vi "Sort moves by minimum incremental travel.vi"(1 "Coordinates to move through":sgl[][](array[numeric])) -> (0 "Indices sorted by minimum incremental travel distance":i32[](array[numeric]))   [LabVIEW 2014]
doc: "Sorts moves in order of minimum incremental linear travel distance, starting from the first point in the list."
uses:
  <vilib>/Analysis/baseanly.llb/Real Dot Product.vi
  <vilib>/Analysis/NI_AALBase.lvlib
panel:
  # "Paul Nathan 02/07/2015"
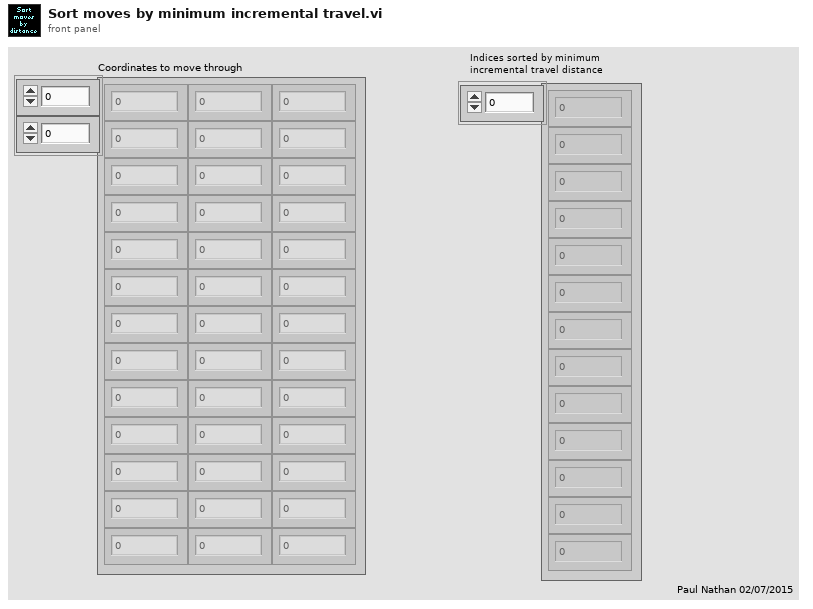
[diagram p1: front panel]
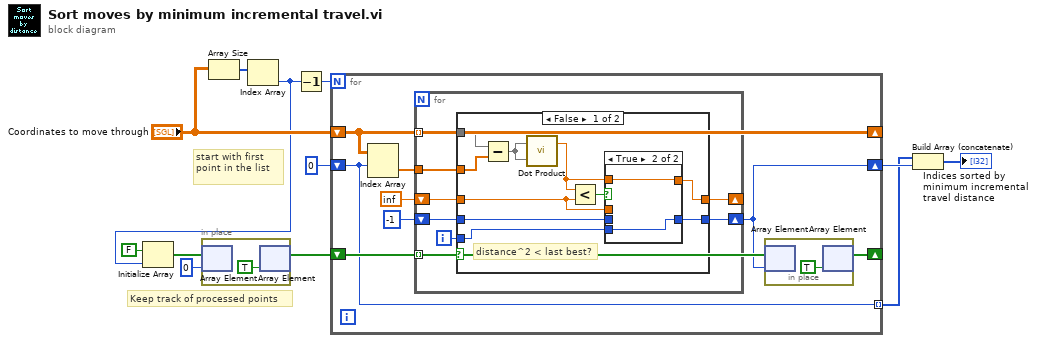
[diagram p0: block diagram]
diagram:
  # "Keep track of processed points"
  # "start with first point in the list"
  n1 = Array Size(array="Coordinates to move through") -> (size(s)=w11:i32[])
  n2 = Index Array(array=w11) -> (element=w9:i32)  [unwired: 1 in]
  n3 = Initialize Array(FALSE, w9) -> (w7:bool[])
  n4 = in-place {
    n5 = in-place-array #1(w7, 0) -> ()  [unwired: 1 out]
    n6 = in-place-array #1(TRUE ("element")) -> (w6:bool[])  [unwired: 1 out]
  }
  n7 = Decrement(x=w9) -> (x-1=w4:i32)
  n8 = for {
    N: w4 -> [_]
    shift-right: [w15] -> _
    shift-left: "Coordinates to move through" -> [w15]
    shift-right: [w19] -> _
    shift-left: w6 -> [w20]
    shift-right: [w16] -> w2
    shift-left: 0 -> [w14]
    tunnel: [w14] -> w1 mode=indexing
    n9 = Index Array(array=w15, index (row)=w14) -> (element=w17:sgl[])  [unwired: 1 in]
    n10 = for {
      tunnel: w15 -> [w30] mode=indexing
      tunnel: w20 -> [w28] mode=indexing
      shift-right: [w24] -> w16
      shift-left: -1 -> [w26]
      shift-right: [w23] -> _
      shift-left: inf ("index (row)") -> [w27]
      tunnel: w17 -> [w29]
      i -> [w25]
      n11 = case shown="False" w28 {
        tunnel: w30 -> [w31 _]
        tunnel: w29 -> [w40 _]
        tunnel: w27 -> [w33 w46]
        tunnel: w26 -> [w32 w45]
        tunnel: w25 -> [w37 _]
        tunnel: [w36 w45] -> w24
        tunnel: [w34 w46] -> w23
        frame False {
          # "distance^2 < last best?"
          n12 = Subtract(x=w31, y=w40) -> (x-y=w39:sgl[])
          n13 = call-poly <vilib>:"Dot Product.vi"("Y Vector"=w39, "X Vector"=w39) -> ("X * Y"=w35:dbl)  [unwired: 1 out]
          n14 = Less?(x=w35, y=w33) -> (x < y?=w38:bool)
          n15 = case shown="True" w38 {
            tunnel: w37 -> [_ w44]
            tunnel: [w41 w44] -> w36
            tunnel: [w42 w43] -> w34
            tunnel: w35 -> [_ w43]
            tunnel: w33 -> [w42 _]
            tunnel: w32 -> [w41 _]
            frame False {
            }
            frame True {
            }
          }
        }
        frame True {
          # "This point already done, skip onto next unprocessed point"
        }
      }
    }
    n16 = in-place {
      n17 = in-place-array #2(w20, w16) -> ()  [unwired: 1 out]
      n18 = in-place-array #2(TRUE ("element")) -> (w19:bool[])  [unwired: 1 out]
    }
  }
  n19 = Build Array (concatenate)(w1, w2) -> (→"Indices sorted by minimum incremental travel distance":i32[])
